vi "Initalize Classes.vi"(8 "error in (no error)":errorcluster, 11 "Channel in":refnum<class "Channel.lvclass">) -> (0 "error out":errorcluster, 3 "Channel out":refnum<class "Channel.lvclass">)   [LabVIEW 2018, in "Channel.lvclass"]
uses:
  Channel.lvclass
  Save Image/Save Image.lvclass
  Channel.lvclass/Channel.ctl
  Simulated_Header/Simulated_Header.lvclass
  CCDCamera/CCDCamera.lvclass
  C:/Users/observer/Desktop/SPARC4_ACS/SPARC4_ACS/Simulated_CCD_Camera/Simulated_CCD_Camera.lvclass
  Header/Header.lvclass
  C:/Users/observer/Desktop/SPARC4_ACS/SPARC4_ACS/Simulated_Header/Simulated_Header.lvclass
panel:
  in  "Save Image in":refnum<class "Save Image.lvclass">
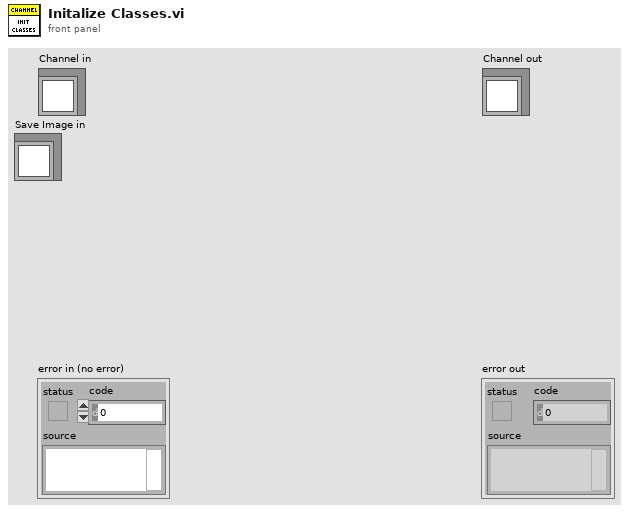
[diagram p1: front panel]
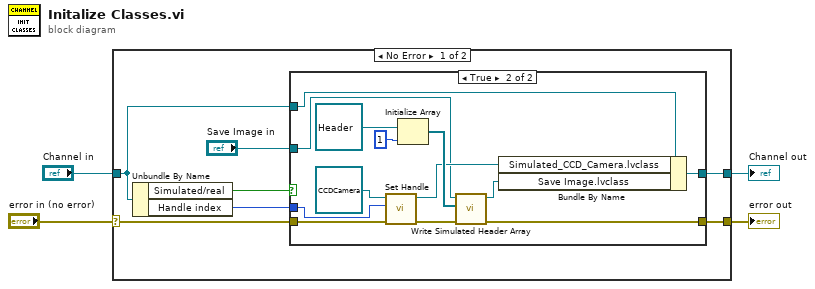
[diagram p0: block diagram]
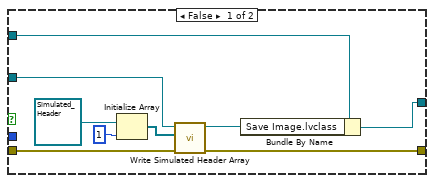
[diagram p2: hidden frame]
diagram:
  n1 = case shown="No Error" "error in (no error)" {
    selector: "error in (no error)" -> [w11 w35]
    tunnel: [w7 w35] -> w3
    tunnel: [w6 w34] -> w1
    tunnel: "Channel in" -> [w8 w34]
    frame No Error {
      n2 = Unbundle By Name(w8) -> ("Simulated/real"=w10:bool, "Handle index"=w9:u16)
      n3 = case shown="True" w10 {
        tunnel: w11 -> [w14 w28]
        tunnel: w9 -> [_ w33]
        tunnel: w8 -> [w17 w26]
        tunnel: [w15 w23] -> w7
        tunnel: [w13 w22] -> w6
        tunnel: "Save Image in" -> [w12 w21]
        frame False {
          n4 = Initialize Array(refnum<class "Simulated_Header.lvclass"> refnum ("Simulated_Header.lvclass"), 1 ("dimension size")) -> (w18:refnum<class "Simulated_Header.lvclass">[])
          n5 = call "Write Simulated Header Array.vi"("error in (no error)"=w14, "Simulated Header Array"=w18, "Save Image in"=w12) -> ("error out"=w15:errorcluster, "Save Image out"=w16:refnum<class "Save Image.lvclass">)  [unwired: 7 in]
          n6 = Bundle By Name(cluster=w17, "Save Image.lvclass"=w16) -> (w13:refnum<class "Channel.lvclass">)
        }
        frame True {
          n7 = call-dynamic "Set Handle.vi"("error in (no error)"=w28, "handle index"=w33, "CCDCamera in"=refnum<class "CCDCamera.lvclass"> refnum ("CCDCamera.lvclass")) -> ("error out"=w27:errorcluster, "CCDCamera out"=w25:refnum<class "CCDCamera.lvclass">)  [unwired: 7 in]
          n8 = Initialize Array(refnum<class "Header.lvclass"> refnum ("Header.lvclass"), 1 ("dimension size")) -> (w30:refnum<class "Header.lvclass">[])
          n9 = call "Write Simulated Header Array.vi"("error in (no error)"=w27, "Simulated Header Array"=w30, "Save Image in"=w21) -> ("error out"=w23:errorcluster, "Save Image out"=w24:refnum<class "Save Image.lvclass">)  [unwired: 7 in]
          n10 = Bundle By Name(cluster=w26, "Simulated_CCD_Camera.lvclass"=w25, "Save Image.lvclass"=w24) -> (w22:refnum<class "Channel.lvclass">)
        }
      }
    }
    frame Error {
    }
  }
  "error out" <- w3
  "Channel out" <- w1
